vi "nanostage-readonly.vi"(4 "error in":errorcluster, 7 "Axes to move":string[](array[string])) -> (0 "error out":errorcluster, 1 "position-z":dbl, 2 "position-y":dbl, 3 "position-x":dbl)   [LabVIEW 2015]
panel:
  # "3D piezo nano stage"
  # "position [µm]"
  # "axis"
  # "x-axis"
  # "y-axis"
  # "z-axis"
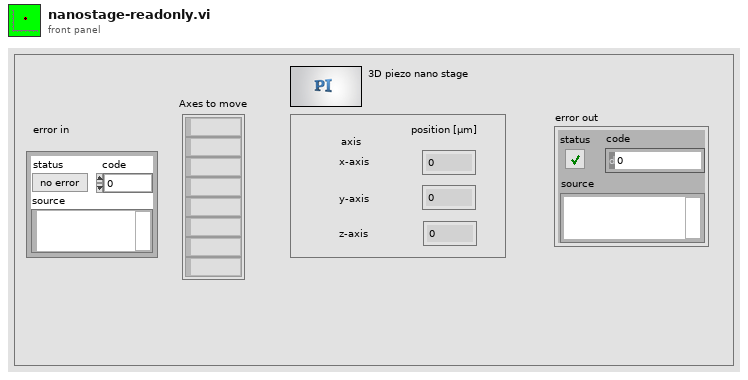
[diagram p1: front panel]
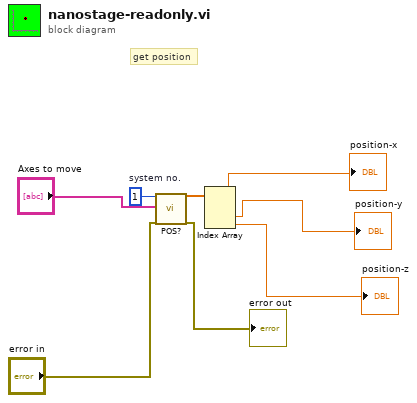
[diagram p0: block diagram]
diagram:
  w5 = 1  # system no.
  # "get position"
  n1 = call "POS?.vi"("System no."=w5, "Axes to query"="Axes to move", "error in"="error in") -> ("Position"=w6:dbl[], "error out"=→"error out":errorcluster)  [unwired: 15 in]
  n2 = Index Array(array=w6) -> (element #1=→"position-x":dbl, element #2=→"position-y":dbl, element #3=→"position-z":dbl)  [unwired: 3 in]
